vi "Write Nested Viewable Enqueuers.vi"(8 "error in (no error)":errorcluster, 9 "Viewable Names (optional)":string[](array[string]), 10 "Nested Viewable Enqueuers":refnum<class "Message Enqueuer.lvclass">[](array[class]), 11 "BoundViewManager In":refnum<class "BoundViewManager.lvclass">) -> (0 "error out":errorcluster, 3 "BoundViewManager Out":refnum<class "BoundViewManager.lvclass">)   [LabVIEW 2020, in "BoundViewManager.lvlib" / "BoundViewManager.lvclass"]
doc: "<License>\nCopyright © 2017 Composed Systems, LLC | All rights reserved\nwww.composed.io\n\nAuthor: Ethan Stern <ethan.stern@composed.io>\n\nThis software is provided \"AS IS\" WITHOUT WARRANTIES, either express or implied, AND IS FOR EDUCATIONAL PURPOSES ONLY.\n</License>"
uses:
  <vilib>/gpm_packages/@cs/ViewManager/source/BoundViewManager/BoundViewManager.lvclass
  <vilib>/ActorFramework/Message Enqueuer/Message Enqueuer.lvclass
  <vilib>/gpm_packages/@cs/ViewManager/source/BoundViewManager/BoundViewManager.lvclass/BoundViewManager.ctl
  <vilib>/gpm_packages/@cs/lookup-table/Source/LookupTable/LookupTable.lvclass/LookupTable.ctl
  092bf4f2-8693-4240-999d-36af2177e143.vi
  <vilib>/gpm_packages/@cs/lookup-table/Source/LookupTable/Read Table Reference.vi
  092bf4f2-8693-4240-999d-36af2177e143.vi/9004466f-827a-42fe-a898-ee956c92e9b7.vi
  <vilib>/gpm_packages/@cs/lookup-table/Source/LookupTable/LookupTable.lvclass
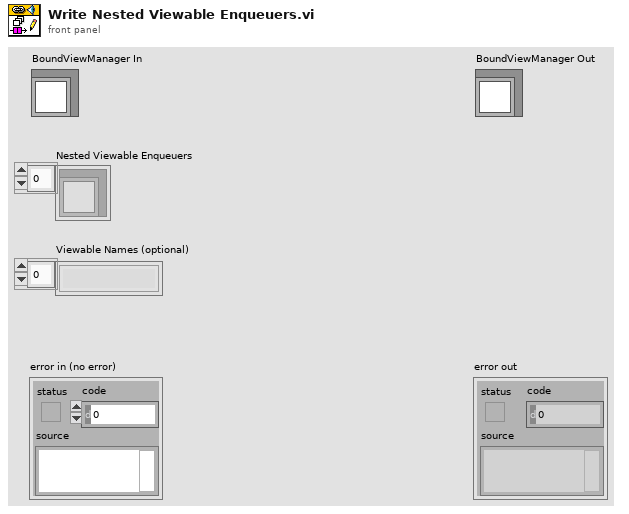
[diagram p1: front panel]
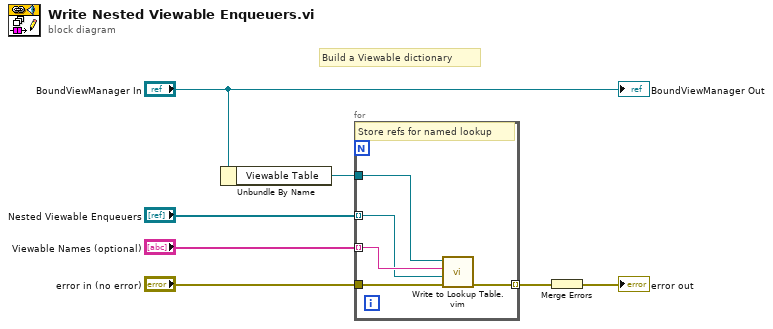
[diagram p0: block diagram]
diagram:
  # "Build a Viewable dictionary"
  n1 = Unbundle By Name("BoundViewManager In") -> ("Viewable Table"=w3:refnum<data-value>)
  n2 = for {
    tunnel: w3 -> [w12]
    tunnel: "Viewable Names (optional)" -> [w11] mode=indexing
    tunnel: "Nested Viewable Enqueuers" -> [w10] mode=indexing
    tunnel: [w9] -> w6 mode=indexing
    tunnel: "error in (no error)" -> [w8]
    # "Store refs for named lookup"
    n3 = call "Write to Lookup Table.vim"("error in (no error)"=w8, "Item"=w10, "Item Name"=w11, "LookupTable Reference"=w12) -> ("error out"=w9:errorcluster)  [unwired: 5 in, 2 out]
  }
  n4 = Merge Errors(w6) -> (→"error out":errorcluster)
  "BoundViewManager Out" <- "BoundViewManager In"
